vi "Write Sender.vi"(10 "Sender":refnum<class "Sender.lvclass">, 11 "Terminated Msg in":refnum<class "Terminated Msg.lvclass">) -> (3 "Terminated Msg out":refnum<class "Terminated Msg.lvclass">)   [LabVIEW 2025, in "jettl.lvlib" / "Terminated Msg.lvlib" / "Terminated Msg.lvclass"]
uses:
  Terminated Msg.lvclass
  Terminated Msg.lvclass/Terminated Msg.ctl
  Sender/Sender/Sender.lvclass
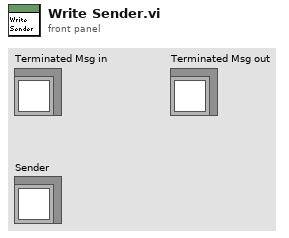
[diagram p1: front panel]
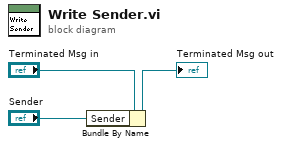
[diagram p0: block diagram]
diagram:
  n1 = Bundle By Name(cluster="Terminated Msg in", "Sender"="Sender") -> (→"Terminated Msg out":refnum<class "Terminated Msg.lvclass">)
